vi "createTelemetry.vi"(8 "error in (no error)":errorcluster, 11 "SAL_Events in":refnum<class "SAL_Events.lvclass">) -> (0 "error out":errorcluster, 3 "SAL_Events out":refnum<class "SAL_Events.lvclass">)   [LabVIEW 2015, in "SAL_Events.lvclass"]
uses:
  SAL_Events.lvclass
  SALLV_domeADB/DataTypes/status.ctl
  SAL_Events.lvclass/SAL_Events.ctl
  SALLV_domeADB/SALLV_domeADB.lvlib
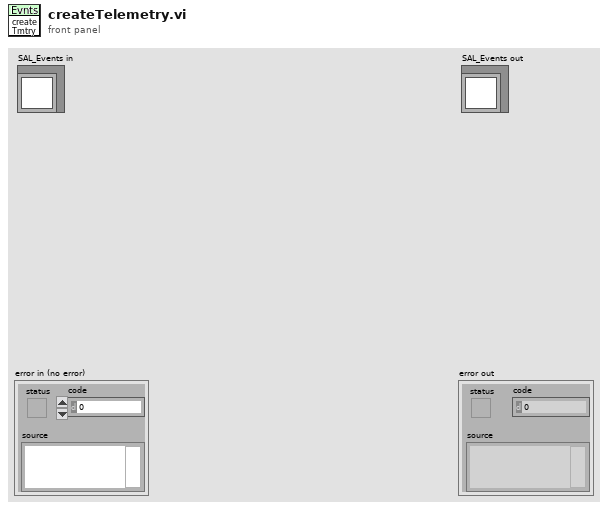
[diagram p1: front panel]
types:
  T1 = typedef "SALLV_domeADB.lvlib/status.ctl" = cluster{"position_error":sgl, "position_actual":sgl, "position_cmd":sgl, "drive_torque_actual[5]":sgl[], "drive_torque_error[5]":sgl[], "drive_torque_cmd[5]":sgl[], "drive_current_actual[5]":sgl[], "drive_temp_actual[5]":sgl[], "encoder_head_raw[5]":sgl[], "encoder_head_calibrated[5]":sgl[], "resolver_raw[5]":sgl[], "resolver_calibrated[5]":sgl[]}
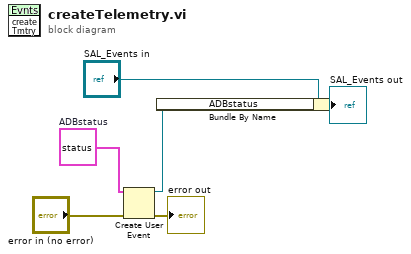
[diagram p0: block diagram]
diagram:
  w6 = T1 {"position_error"=0.0, "position_actual"=0.0, "position_cmd"=0.0, "drive_torque_actual[5]"=[0.0, 0.0, 0.0, 0.0, 0.0], "drive_torque_error[5]"=[0.0, 0.0, 0.0, 0.0, 0.0], "drive_torque_cmd[5]"=[0.0, 0.0, 0.0, 0.0, 0.0], "drive_current_actual[5]"=[0.0, 0.0, 0.0, 0.0, 0.0], "drive_temp_actual[5]"=[0.0, 0.0, 0.0, 0.0, 0.0], "encoder_head_raw[5]"=[0.0, 0.0, 0.0, 0.0, 0.0], "encoder_head_calibrated[5]"=[0.0, 0.0, 0.0, 0.0, 0.0], "resolver_raw[5]"=[0.0, 0.0, 0.0, 0.0, 0.0], "resolver_calibrated[5]"=[0.0, 0.0, 0.0, 0.0, 0.0]}  # ADBstatus
  n1 = Create User Event(user event datatype=w6, error in="error in (no error)") -> (user event=w2:refnum<user-event>, error out=→"error out":errorcluster)
  n2 = Bundle By Name(cluster="SAL_Events in", "ADBstatus"=w2) -> (→"SAL_Events out":refnum<class "SAL_Events.lvclass">)
